vi "Get Measurement Details.vi"(8 "error in":errorcluster) -> (0 "error out":errorcluster, 2 "Service ID":string caption="service_class", 3 "measurement_details":T1)   [LabVIEW 2020, in "LoadRegulation.lvlib"]
uses:
  LoadRegulation.lvlib
  RPC Messages/ni_measurements_v1_MeasurementDetails.ctl
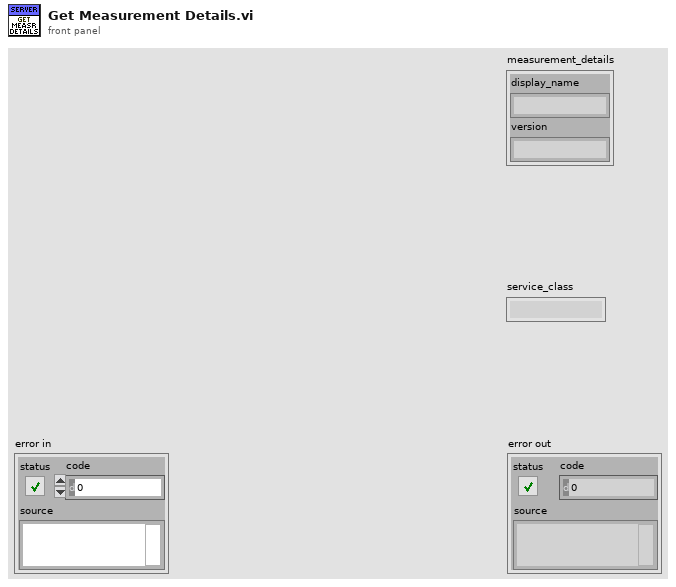
[diagram p1: front panel]
types:
  T1 = typedef "LoadRegulation.lvlib/ni_measurements_v1_MeasurementDetails.ctl" = cluster{"display_name":string, "version":string}
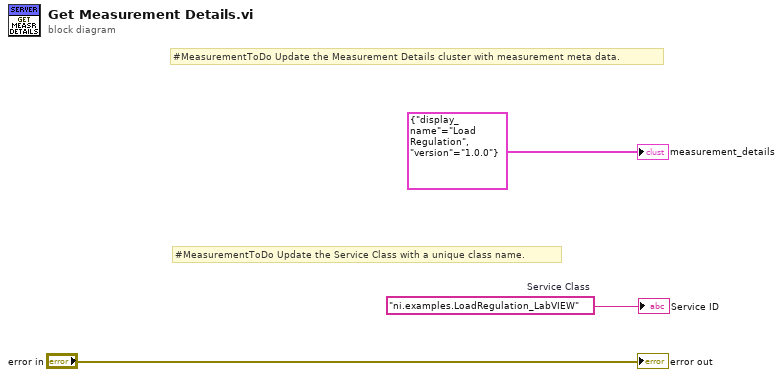
[diagram p0: block diagram]
diagram:
  w1 = "ni.examples.LoadRegulation_LabVIEW"  # Service Class
  # "#MeasurementToDo Update the Service Class with a unique class name."
  # "#MeasurementToDo Update the Measurement Details cluster with measurement meta data."
  "error out" <- "error in"
  "measurement_details" <- T1 {"display_name"="Load Regulation", "version"="1.0.0"} ("measurement_details")
  "Service ID" <- w1
